vi "Carney_exercise1.vi"   [LabVIEW 2014, in "Carney_exercise1.lvrbt"]
uses:
  Carney_exercise1.lvrbt
  <vilib>/NXT/Block Support/NXT_OutputPort.ctl
  <vilib>/NXT/NXTIO Xnodes/NXTIONodeSubVIs/NXTMoveMotors.vi
  <vilib>/NXT/Dual Mode Library/Waits/Wait_Num.vi
  <vilib>/NXT/Subs/LVHSConnector.ctl
  <vilib>/NXT/NXTIO Xnodes/AddressXNode/NXTIOAddress.xnode
  <vilib>/NXT/NXTIO Xnodes/NXTIOXNode/NXTIO.xnode
  <vilib>/NXT/LegoClasses/BrickReference/BrickReference.lvclass
types:
  T1 = typedef "NXT_OutputPort.ctl" = u8
  T2 = typedef "LVHSConnector.ctl" = refnum<class "BrickReference.lvclass">
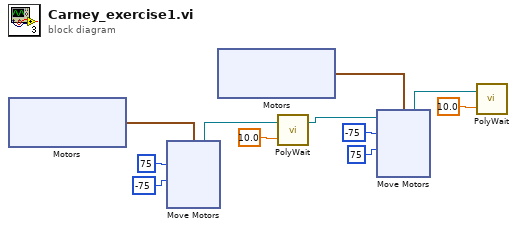
[diagram p0: block diagram]
diagram:
  n1 = xnode "Motors"() -> ("Motor"=w11:cluster{"Port":T1, "Port":T1})
  n2 = xnode "Move Motors"("Power/Speed 2"=i8 -75, "Power/Speed 1"=i8 75, "Motors"=w11) -> ("NXT/EV3"=w7:T2)  [unwired: 1 in]
  n3 = xnode "Motors"() -> ("Motor"=w6:cluster{"Port":T1, "Port":T1})
  n4 = call-poly <vilib>:"PolyWait.vi"("Time (1 sec)"=sgl 10.0, "NXT/EV3"=w7) -> ("NXT/EV3"=w1:T2)  [unwired: 2 in]
  n5 = xnode "Move Motors"("Power/Speed 2"=i8 75, "Power/Speed 1"=i8 -75, "Motors"=w6, "NXT/EV3"=w1) -> ("NXT/EV3"=w2:T2)
  n6 = call-poly <vilib>:"PolyWait.vi"("Time (1 sec)"=sgl 10.0, "NXT/EV3"=w2) -> ()  [unwired: 2 in, 1 out]
